vi "DiodeTest.vi"(4 "Stimulus_LED":refnum<vi>, 5 "Peltier_OnOffs":refnum<vi>, 6 "DelayStr Ref":refnum<vi>, 7 "Abort Ref":refnum<vi>, 8 "error in (no error)":errorcluster, 11 "CurrentTest":T1 {"Post-Log(s)" format="%#_13g"; "Pre-Log (s)" format="%#_13g"; "Duration (s)" format="%#_13g"}) -> (0 "error out":errorcluster)   [LabVIEW 2025]
uses:
  controls/SingleTest.ctl
  controls/TestType.ctl
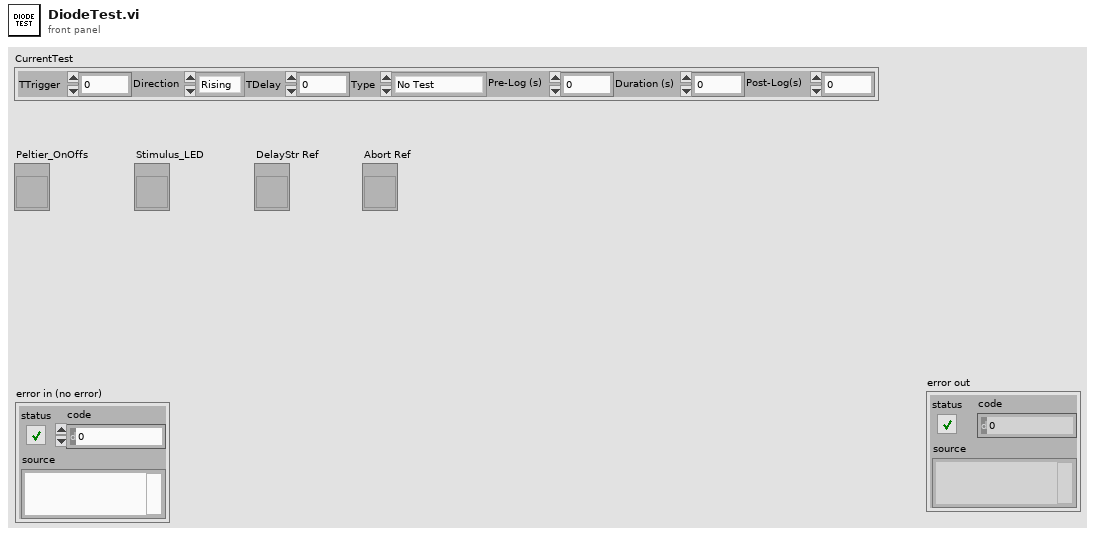
[diagram p1: front panel]
types:
  T1 = typedef "SingleTest.ctl" = cluster{"TTrigger":dbl, "Direction":enum16{"Rising", "Falling"}, "TDelay":dbl, "Type":T2, "Pre-Log (s)":dbl, "Duration (s)":dbl, "Post-Log(s)":dbl}
  T2 = typedef "TestType.ctl" = enum16{"No Test", "Heater Test", "Actuation Test", "Diode Test"}
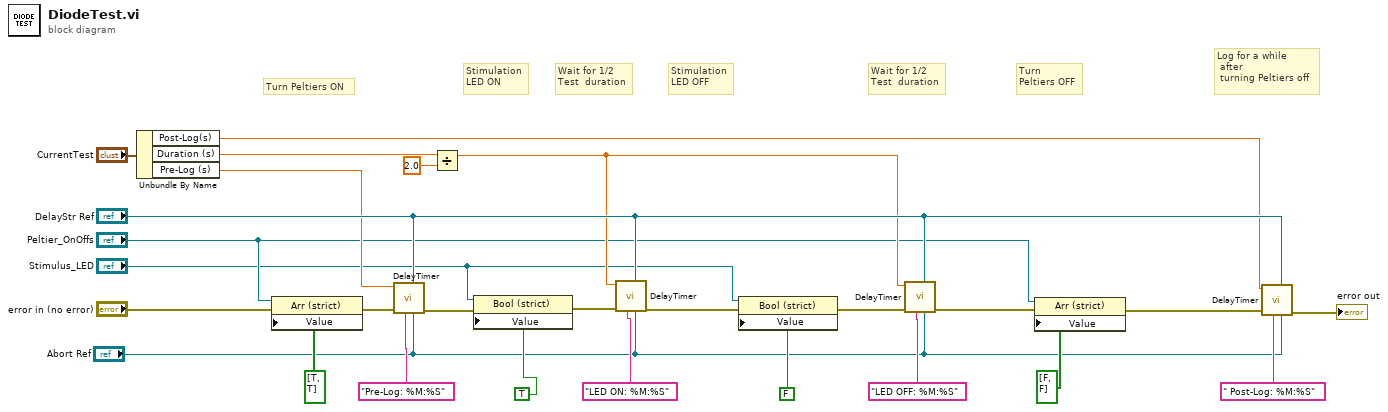
[diagram p0: block diagram]
diagram:
  # "Stimulation\nLED OFF"
  # "Wait for 1/2 \nTest  duration"
  # "Stimulation\nLED ON"
  # "Log for a while\n after\n turning Peltiers off"
  # "Wait for 1/2 \nTest  duration"
  # "Turn \nPeltiers OFF"
  # "Turn Peltiers ON"
  n1 = Unbundle By Name("CurrentTest") -> ("Post-Log(s)"=w14:dbl, "Duration (s)"=w13:dbl, "Pre-Log (s)"=w12:dbl)
  n2 = property on="Property Node" class="Arr (strict)"(reference="Peltier_OnOffs", error in="error in (no error)", "Value"=bool[] [TRUE, TRUE]) -> (error out=w25:errorcluster)  [unwired: 1 out]
  n3 = call "DelayTimer.vi"("Abort Ref"="Abort Ref", "Formatted \nTime Ref"="DelayStr Ref", "FormatString"="Pre-Log: %M:%S", "error in (no error)"=w25, "Delay(s)"=w12) -> ("error out"=w26:errorcluster)  [unwired: 6 in]
  n4 = Divide(x=w13, y=2.0) -> (x/y=w22:dbl)
  n5 = property on="Property Node" class="Bool (strict)"(reference="Stimulus_LED", error in=w26, "Value"=TRUE ("LED_Stimulate")) -> (error out=w16:errorcluster)  [unwired: 1 out]
  n6 = call "DelayTimer.vi"("Abort Ref"="Abort Ref", "Formatted \nTime Ref"="DelayStr Ref", "FormatString"="LED ON: %M:%S", "error in (no error)"=w16, "Delay(s)"=w22) -> ("error out"=w18:errorcluster)  [unwired: 6 in]
  n7 = property on="Property Node" class="Bool (strict)"(reference="Stimulus_LED", error in=w18, "Value"=FALSE ("LED_Stimulate")) -> (error out=w21:errorcluster)  [unwired: 1 out]
  n8 = call "DelayTimer.vi"("Abort Ref"="Abort Ref", "Formatted \nTime Ref"="DelayStr Ref", "FormatString"="LED OFF: %M:%S", "error in (no error)"=w21, "Delay(s)"=w22) -> ("error out"=w20:errorcluster)  [unwired: 6 in]
  n9 = property on="Property Node" class="Arr (strict)"(reference="Peltier_OnOffs", error in=w20, "Value"=bool[] [FALSE, FALSE]) -> (error out=w5:errorcluster)  [unwired: 1 out]
  n10 = call "DelayTimer.vi"("Abort Ref"="Abort Ref", "Formatted \nTime Ref"="DelayStr Ref", "FormatString"=" Post-Log: %M:%S", "error in (no error)"=w5, "Delay(s)"=w14) -> ("error out"=→"error out":errorcluster)  [unwired: 6 in]
